vi "LibXML_QueryXPathExpr.vi"(8 "error in":errorcluster, 9 "rootnode (root of doc)":u32, 10 "XPathExpr":string="/ScanMaster/Devices/Device/description", 11 "doc":u32) -> (0 "error out":errorcluster, 3 "xmlXPathObj":u32)   [LabVIEW 2019, in "Tools.lvlib" / "LibXML.lvlib"]
doc: "NOTE: rootnode (root of doc) is the node relative to which RELATIVE XPath expressions\nare evaluated. relative XPath expressions do NOT start\nwith s slash = \"/\".\nIf rootnode=0, then the document root node is used\nas starting point for relative expressions"
uses:
  LibXML.lvlib
  <vilib>/Utility/error.llb/Trim Whitespace.vi
  Tools.lvlib
  dll/lXMLwrap.dll
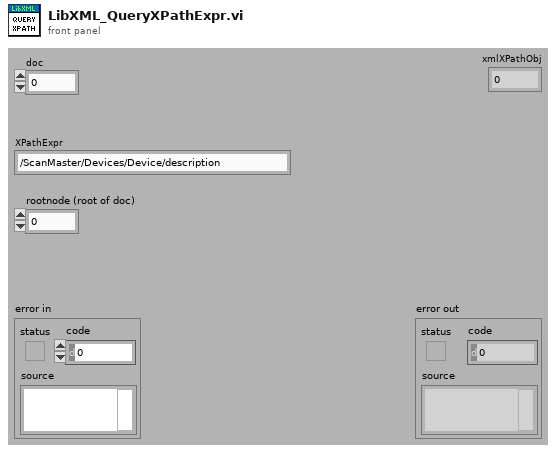
[diagram p1: front panel]
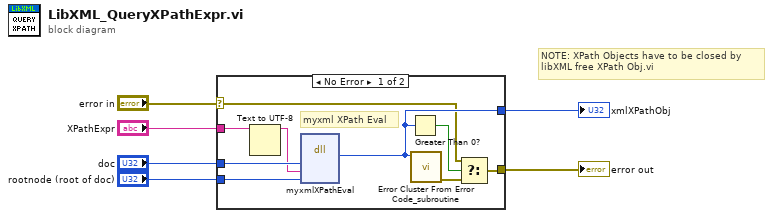
[diagram p0: block diagram]
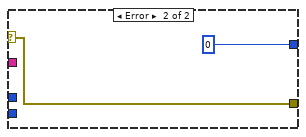
[diagram p2: hidden frame]
diagram:
  # "NOTE: XPath Objects have to be closed by\nlibXML free XPath Obj.vi"
  n1 = case shown="No Error" "error in" {
    selector: "error in" -> [w9 w17]
    tunnel: [w14 w17] -> w5
    tunnel: [w12 u32 0] -> w4
    tunnel: "XPathExpr" -> [w8 _]
    tunnel: "doc" -> [w11 _]
    tunnel: "rootnode (root of doc)" -> [w10 _]
    frame No Error {
      # "myxml XPath Eval"
      n2 = Text to UTF-8(11:w8) -> (3:w7:string)  [unwired: 2 in, 1 out]
      n3 = dll-call lib="C:/Projects/_Prywatne/MyCIT/Framework/Tools/XML/LibXML/dll/lXMLwrap.dll" fn="myxmlXPathEval"("doc"=w11, "xpathexpr"=w7, "rootnode"=w10) -> ("return type"=w12:u32)  [unwired: 6 in, 2 out]
      n4 = Greater Than 0?(x=w12) -> (x > 0?=w15:bool)
      n5 = call "Error Cluster From Error Code_subroutine.vi"("error code (0)"=w12) -> ("error out"=w13:errorcluster)  [unwired: 8 in]
      n6 = Select(t=w9, s=w15, f=w13) -> (s? t:f=w14:errorcluster)
    }
    frame Error {
    }
  }
  "error out" <- w5
  "xmlXPathObj" <- w4
